vi "read_H2_N2.vi"() -> (0 "H2N2 Flow Rate":dbl, 1 "H2N2 Remote":bool, 2 "Display H2N2":bool, 3 "N2 Active":bool, 4 "H2 Active":bool)   [LabVIEW 2011]
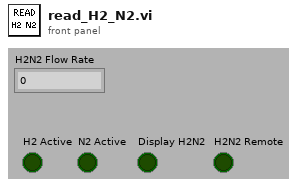
[diagram p1: front panel]
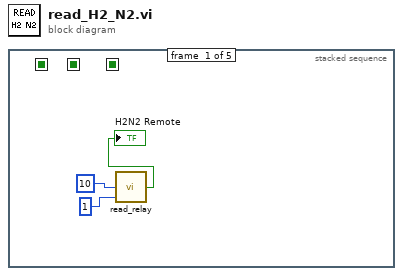
[diagram p0: block diagram]
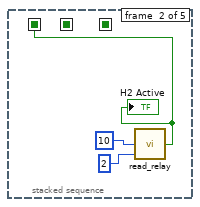
[diagram p2: hidden frame]
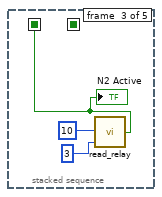
[diagram p3: hidden frame]
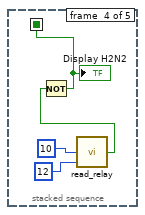
[diagram p4: hidden frame]
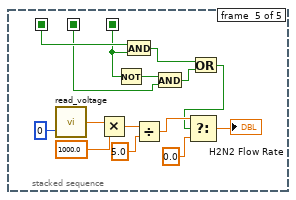
[diagram p5: hidden frame]
diagram:
  n1 = stacked-sequence {
    seq-local: [_ w4 _ _ _] -> [_ _ _ _ w20]
    seq-local: [_ _ w7 _ _] -> [_ _ _ _ w18]
    seq-local: [_ _ _ w10 _] -> [_ _ _ _ w19]
    frame #0 {
      n2 = call "read_relay.vi"("Relay"=1, "Slot"=10) -> ("Relay Status"=→"H2N2 Remote":bool)  [unwired: 1 out]
    }
    frame #1 {
      n3 = call "read_relay.vi"("Relay"=2, "Slot"=10) -> ("Relay Status"=w4:bool)  [unwired: 1 out]
      "H2 Active" <- w4
    }
    frame #2 {
      n4 = call "read_relay.vi"("Relay"=3, "Slot"=10) -> ("Relay Status"=w7:bool)  [unwired: 1 out]
      "N2 Active" <- w7
    }
    frame #3 {
      n5 = call "read_relay.vi"("Relay"=12, "Slot"=10) -> ("Relay Status"=w11:bool)  [unwired: 1 out]
      n6 = Not(x=w11) -> (.not. x?=w10:bool)
      "Display H2N2" <- w10
    }
    frame #4 {
      n7 = call "read_voltage.vi"("Channel"=0) -> ("Voltage"=w27:dbl)  [unwired: 1 in]
      n8 = Multiply(x=w27, y=1000.0) -> (x*y=w25:dbl)
      n9 = Not(x=w19) -> (.not. x?=w17:bool)
      n10 = And(x=w20, y=w19) -> (x .and. y?=w16:bool)
      n11 = Divide(x=w25, y=5.0) -> (x/y=w23:dbl)
      n12 = And(x=w17, y=w18) -> (x .and. y?=w15:bool)
      n13 = Or(x=w16, y=w15) -> (x .or. y?=w14:bool)
      n14 = Select(t=w23, s=w14, f=0.0) -> (s? t:f=→"H2N2 Flow Rate":dbl)
    }
  }
